vi "Pendulum time Since Timer Start u S.vi"() -> (3 "function return":dbl)   [LabVIEW 2024, in "pendulumApp.lvlib"]
doc: "OOTB_API double Pendulum_timeSinceTimerStart_uS();"
uses:
  pendulumApp.lvlib
  pendulumApp.dll
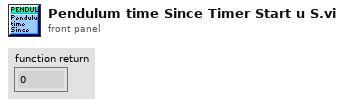
[diagram p1: front panel]
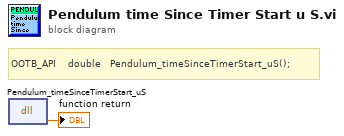
[diagram p0: block diagram]
diagram:
  # "OOTB_API    double   Pendulum_timeSinceTimerStart_uS();"
  n1 = dll-call lib="C:/Users/scer/OneDrive - University of Florida/eml4314c/eml4314cFA25/Resources/FA25_dev_version2/SADI_Pendulum_lib/pendulumApp.*" fn="Pendulum_timeSinceTimerStart_uS"() -> (→"function return":dbl)  [unwired: 3 in, 2 out]
